vi "Drive Control (SubVI).vi"(8 "Buttons":bool[](array[boolean]), 9 "Joystick Axis":dbl[](array[numeric]), 10 "PID gains Slow":T1={"proportional gain (Kc)"=0.7500000000000001, "integral time (Ti, min)"=0.004, "derivative time (Td, min)"=0.0} {"derivative time (Td, min)" format="%.3f"; "integral time (Ti, min)" format="%.3f"; "proportional gain (Kc)" format="%.3f"}, 11 "PID gains Fast":T1={"proportional gain (Kc)"=0.7500000000000001, "integral time (Ti, min)"=0.001, "derivative time (Td, min)"=0.0} {"derivative time (Td, min)" format="%.3f"; "integral time (Ti, min)" format="%.3f"; "proportional gain (Kc)" format="%.3f"}) -> ()   [LabVIEW 2014]
uses:
  <vilib>/Rock Robotics/WPI/RobotDrive/WPI_RobotDriveGetSetRefNum.vi
  <vilib>/addons/control/pid/pid.llb/PID Control Input Filter (DBL).vi
  <vilib>/addons/control/pid/pid.llb/PID (DBL).vi
  <vilib>/Rock Robotics/Network Tables/SD Write Numeric Array.vi
  <vilib>/addons/control/pid/NI_PID_pid.lvlib
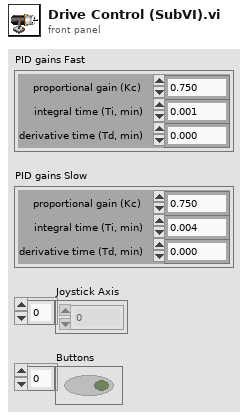
[diagram p1: front panel]
types:
  T1 = cluster{"proportional gain (Kc)":dbl, "integral time (Ti, min)":dbl, "derivative time (Td, min)":dbl}
  T2 = typedef "WPI_RobotDriveDevRef.ctl" = cluster{"DevStatus":errorcluster, "Motors[]":T3[], "Square Inputs":bool, "Max Output":dbl}
  T3 = typedef "WPI_MotorControlDeviceRef.ctl" = cluster{"DeviceStatus":errorcluster, "Type":T4, "PWM":cluster{"Controller":T5, "PWM Channel":T6, "DeadBand":T7}, "CAN":cluster{"Device Number":u8, "Control Mode":T8, "Semaphore":T9, "Max Vout":dbl, "TalonSRX Control Mode":T10}, "Invert":bool, "TransformRef":T11, "InvTransformRef":T11}
  T4 = typedef "WPI_MotorControlType.ctl" = enum16{"PWM", "CAN", "CANTalonSRX"}
  T5 = typedef "FPGA_TypedefDigitalModule.ctl" = enum16{"Controller 1"}
  T6 = typedef "FPGA_DIOPWMChannel.ctl" = enum8{"PWM 0", "PWM 1", "PWM 2", "PWM 3", "PWM 4", "PWM 5", "PWM 6", "PWM 7", "PWM 8", "PWM 9", "PWM MXP 0", "PWM MXP 1", "PWM MXP 2", "PWM MXP 3", "PWM MXP 4", "PWM MXP 5", "PWM MXP 6", "PWM MXP 7", "PWM MXP 8", "PWM MXP 9", "Invalid"}
  T7 = typedef "WPI_PWMDeadband.ctl" = cluster{"Name":string, "maxPositivePwm":i32, "minPositivePwm":i32, "centerPwm":i32, "maxNegativePwm":i32, "minNegativePwm":i32, "angularRange":u16}
  T8 = typedef "WPI_CANJaguar_ControlMode.ctl" = enum8{"Percent VBus", "Current", "Speed", "Position", "Voltage"}
  T9 = typedef "Semaphore RefNum" = refnum<k1>
  T10 = typedef "WPI_CANTalonSRX_APIControlMode.ctl" = enum8{"Percent VBus", "Speed", "Position", "Slave", "Unchanged / Invalid"}
  T11 = typedef "WPI_PWMTransform_ConPane.ctl" = refnum<vi>
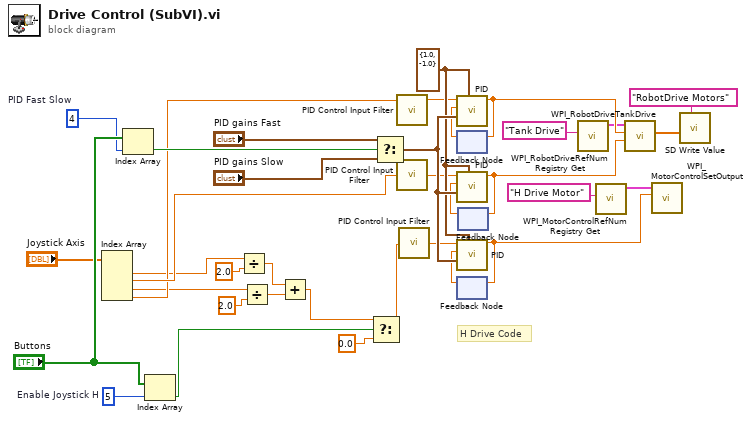
[diagram p0: block diagram]
diagram:
  w34 = 4  # PID Fast Slow
  w32 = 5  # Enable Joystick H
  w25 = cluster{"output high":dbl, "output low":dbl} {"output high"=1.0, "output low"=-1.0} ("output range")
  # "H Drive Code"
  n1 = Index Array(array="Joystick Axis") -> (element #1=w5:dbl, element #2=w31:dbl, element #3=w6:dbl, element #4=w22:dbl)  [unwired: 4 in]
  n2 = Index Array ("H Drive Triggers")(array="Buttons", index=w34) -> (element=w36:bool)
  n3 = Index Array ("H Drive Triggers")(array="Buttons", index=w32) -> (element=w33:bool)
  n4 = Divide(x=w5, y=2.0) -> (x/y=w9:dbl)
  n5 = Divide(x=w6, y=2.0) -> (x/y=w7:dbl)
  n6 = Add(x=w9, y=w7) -> (x+y=w26:dbl)
  n7 = Select(t=w26, s=w33, f=0.0) -> (s? t:f=w28:dbl)
  n8 = Select(t="PID gains Fast", s=w36, f="PID gains Slow") -> (s? t:f=w27:T1)
  n9 = call-poly <vilib>:"PID Control Input Filter.vi"("input"=w22) -> ("output"=w16:dbl)  [unwired: 4 in]
  n10 = call-poly <vilib>:"PID Control Input Filter.vi"("input"=w31) -> ("output"=w15:dbl)  [unwired: 4 in]
  n11 = call-poly <vilib>:"PID Control Input Filter.vi"("input"=w28) -> ("output"=w23:dbl)  [unwired: 4 in]
  n12 = feedback #1() -> (w17:dbl)  [unwired: 1 in]
  n13 = call-poly <vilib>:"PID.vi"("output range"=w25, "PID gains"=w27, "process variable"=w17, "setpoint"=w16) -> ("output"=w18:dbl)  [unwired: 6 in, 1 out]
  n14 = feedback-in #1(w18) -> ()
  n15 = feedback #2() -> (w24:dbl)  [unwired: 1 in]
  n16 = call-poly <vilib>:"PID.vi"("output range"=w25, "PID gains"=w27, "process variable"=w24, "setpoint"=w23) -> ("output"=w29:dbl)  [unwired: 6 in, 1 out]
  n17 = feedback-in #2(w29) -> ()
  n18 = feedback #3() -> (w14:dbl)  [unwired: 1 in]
  n19 = call-poly <vilib>:"PID.vi"("output range"=w25, "PID gains"=w27, "process variable"=w14, "setpoint"=w15) -> ("output"=w19:dbl)  [unwired: 6 in, 1 out]
  n20 = feedback-in #3(w19) -> ()
  n21 = call <vilib>:"WPI_RobotDriveRefNum Registry Get.vi"("refnum name"="Tank Drive") -> ("RobotDriveDevRef"=w13:T2)  [unwired: 1 in, 9 out]
  n22 = call <vilib>:"WPI_MotorControlRefNum Registry Get.vi"("refnum name"="H Drive Motor") -> ("MotorControlDevRef"=w11:T3)  [unwired: 9 in, 1 out]
  n23 = call <vilib>:"WPI_RobotDriveTankDrive.vi"("Right axis value"=w19, "Left axis value"=w18, "RobotDriveDevRef"=w13) -> ("Motor Values"=w4:dbl[])  [unwired: 6 in, 2 out]
  n24 = call <vilib>:"WPI_MotorControlSetOutput.vi"("Output"=w29, "MotorControlDevRef"=w11) -> ()  [unwired: 7 in, 3 out]
  n25 = call-poly <vilib>:"SD Write Value.vi"("Numeric Array"=w4, "Name"="RobotDrive Motors") -> ()  [unwired: 8 in, 2 out]
